vi "destroy.vi"(8 "error in (no error)":errorcluster, 11 "system.logging in":refnum<class "system.logging.lvclass">) -> (0 "error out":errorcluster)   [LabVIEW 2021, in "system.logging.lvclass"]
uses:
  system.logging.lvclass
  system.logging.lvclass/system.logging.ctl
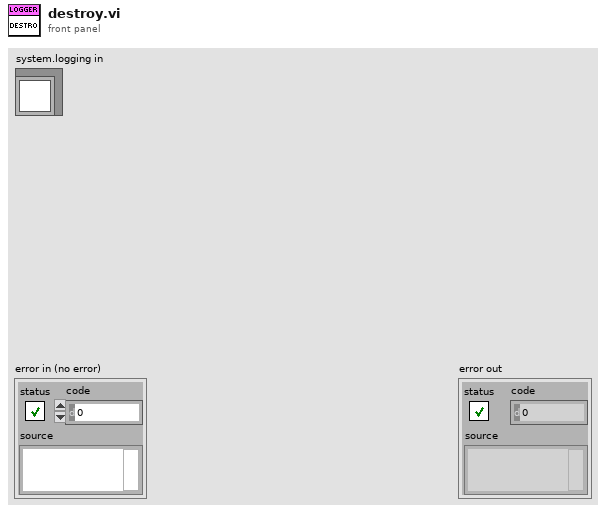
[diagram p1: front panel]
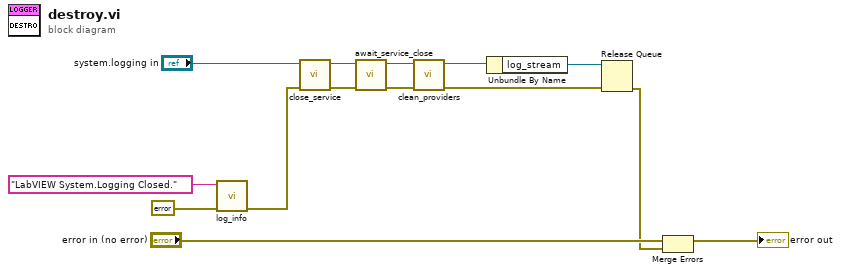
[diagram p0: block diagram]
diagram:
  n1 = call "log_info.vi"("error in (no error)"=errorcluster {"status"=FALSE, "code"=0, "source"=""}, "message"="LabVIEW System.Logging Closed.") -> ("error out"=w9:errorcluster)  [unwired: 9 in]
  n2 = call "close_service.vi"("error in (no error)"=w9, "system.logging (in)"="system.logging in") -> ("error out"=w7:errorcluster, "system.logging (out)"=w8:refnum<class "system.logging.lvclass">)  [unwired: 8 in]
  n3 = call "await_service_close.vi"("error in (no error)"=w7, "system.logging in"=w8) -> ("error out"=w5:errorcluster, "system.logging out"=w6:refnum<class "system.logging.lvclass">)  [unwired: 8 in]
  n4 = call "clean_providers.vi"("error in (no error)"=w5, "system.logging in"=w6) -> ("error out"=w2:errorcluster, "system.logging out"=w4:refnum<class "system.logging.lvclass">)  [unwired: 8 in]
  n5 = Unbundle By Name(w4) -> ("log_stream"=w3:refnum<queue>)
  n6 = Release Queue(queue=w3, error in (no error)=w2) -> (error out=w1:errorcluster)  [unwired: 1 in, 2 out]
  n7 = Merge Errors("error in (no error)", w1) -> (→"error out":errorcluster)
